vi "Generate Signal.vi"(8 "error in (no error)":errorcluster, 9 "Amplitude (1)":dbl=0.5, 10 "Frequency (1000 Hz)":dbl=1000.0, 11 "AgSigGen in":refnum<class "Ag Sig Gen.lvclass">) -> (0 "error out":errorcluster, 3 "AgSigGen out":refnum<class "Ag Sig Gen.lvclass">)   [LabVIEW 2010, in "Ag Sig Gen.lvclass"]
uses:
  Ag Sig Gen.lvclass
  Ag Sig Gen.lvclass/Ag Sig Gen.ctl
panel:
  in  "Waveform Function (1: Sine)":u16(ring)=1 items=["DC", "Sine", "Square", "Triangle", "Ramp", "Pulse", "Noise", "Sinc", "Negative Ramp", "Exponential Rise", "Exponential Fall", "Cardiac"]
  # "For some reason, the actual peak-to-peak read by the tek scope is 2X amplitude"
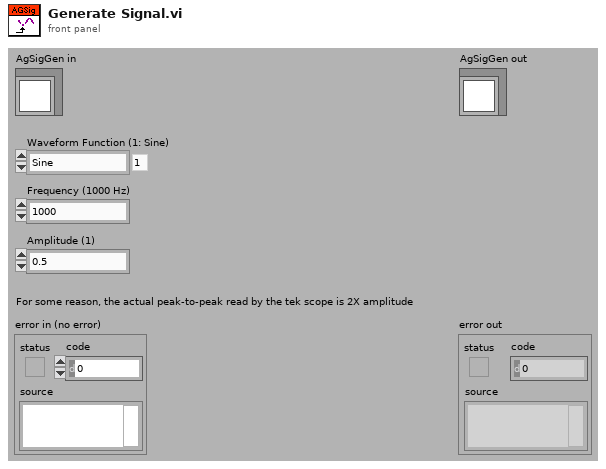
[diagram p1: front panel]
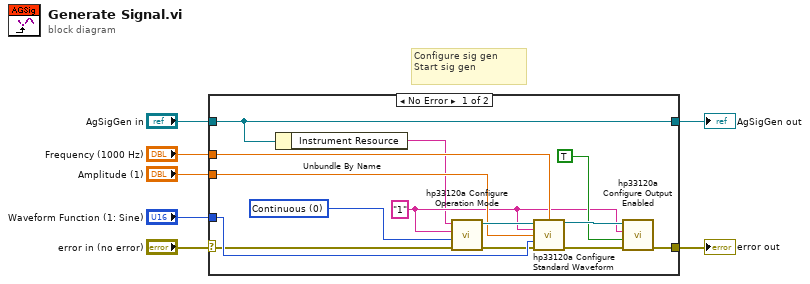
[diagram p0: block diagram]
diagram:
  # "Configure sig gen\nStart sig gen"
  n1 = case shown="No Error" "error in (no error)" {
    selector: "error in (no error)" -> [w10 w23]
    tunnel: [w12 w23] -> w7
    tunnel: "AgSigGen in" -> [w9 w22]
    tunnel: [w9 w22] -> w6
    tunnel: "Amplitude (1)" -> [w17 _]
    tunnel: "Waveform Function (1: Sine)" -> [w16 _]
    tunnel: "Frequency (1000 Hz)" -> [w18 _]
    frame No Error {
      w21 = 0 items=["Continuous"=0, "Burst"=1, "Gate"=1001, "Sweep"=1002] ("operation mode (Continuous)")
      w11 = "1" ("channel name (\"1\")")
      n2 = Unbundle By Name(w9) -> ("Instrument Resource"=w8:string)
      n3 = call <instrlib>:"hp33120a Configure Operation Mode.vi"("error in (no error)"=w10, "operation mode (Continuous)"=w21, "channel name (\"1\")"=w11, "Instrument Handle"=w8) -> ("error out"=w15:errorcluster, "Instrument Handle out"=w19:refnum<k15>)  [unwired: 6 out]
      n4 = call <instrlib>:"hp33120a Configure Standard Waveform.vi"("Instrument Handle"=w19, "frequency (1000.0 Hz)"=w18, "channel name (\"1\")"=w11, "amplitude (0.10 Vpp)"=w17, "waveform (1: Sine)"=w16, "error in (no error)"=w15) -> ("Instrument Handle out"=w20:refnum<k15>, "error out"=w14:errorcluster)  [unwired: 2 in, 6 out]
      n5 = call <instrlib>:"hp33120a Configure Output Enabled.vi"("error in (no error)"=w14, "output enabled (True)"=TRUE ("Enable Output  (T: Enable)"), "channel name (\"1\")"=w11, "Instrument Handle"=w20) -> ("error out"=w12:errorcluster)  [unwired: 7 out]
    }
    frame Error {
    }
  }
  "error out" <- w7
  "AgSigGen out" <- w6
